vi "Receive Messenger.vi"(8 "error in (no error)":errorcluster, 10 "Messenger In":refnum<class "Messenger.lvclass">, 11 "Node Actor in":refnum<class "Node Actor.lvclass">) -> (0 "error out":errorcluster, 3 "Node Actor out":refnum<class "Node Actor.lvclass">)   [LabVIEW 2024, in "Node Actor.lvclass"]
uses:
  Node Actor.lvclass
  Node Actor.lvclass/Node Actor.ctl
  Messenger/Messenger/Messenger.lvclass
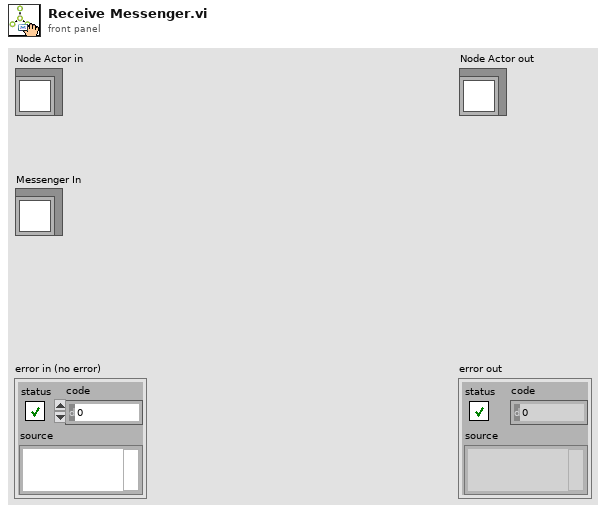
[diagram p1: front panel]
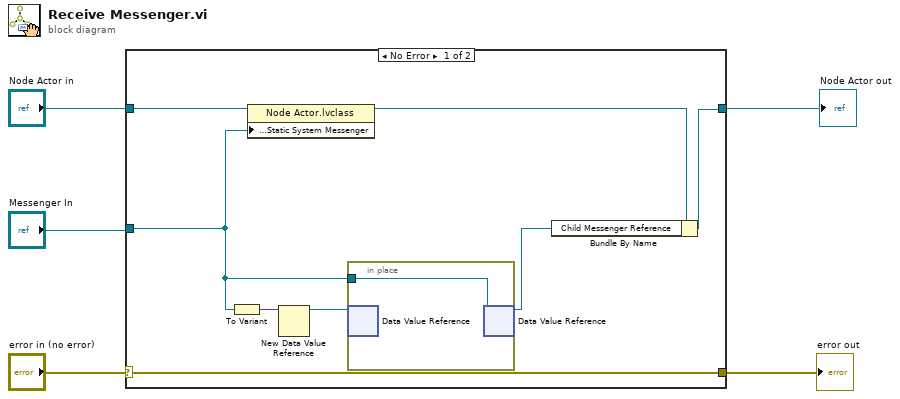
[diagram p0: block diagram]
diagram:
  n1 = case shown="No Error" "error in (no error)" {
    selector: "error in (no error)" -> [w13 w16]
    tunnel: [w13 w16] -> w4
    tunnel: [w10 w15] -> w1
    tunnel: "Node Actor in" -> [w8 w15]
    tunnel: "Messenger In" -> [w6 _]
    frame No Error {
      n2 = To Variant(anything=w6) -> (Variant=w12:variant)
      n3 = property class="Node Actor.lvclass"(reference=w8, "Protected Data:Static System Messenger"=w6) -> (reference out=w7:refnum<class "Node Actor.lvclass">)  [unwired: 1 in, 1 out]
      n4 = New Data Value Reference(data value=w12) -> (data value reference=w11:refnum<data-value>)  [unwired: 1 in, 1 out]
      n5 = in-place {
        in-place-border: w6 -> [w14]
        n6 = in-place-dvr #1(w11) -> ()  [unwired: 2 out]
        n7 = in-place-dvr #1(w14) -> (w9:refnum<data-value>)  [unwired: 1 out]
      }
      n8 = Bundle By Name(cluster=w7, "Child Messenger Reference"=w9) -> (w10:refnum<class "Node Actor.lvclass">)
    }
    frame Error {
    }
  }
  "error out" <- w4
  "Node Actor out" <- w1
